vi "DAQmx 9411 6ch Digital Input (SubVI).vi"(0 "9411 Name":tag="9411", 11 "Error Input":errorcluster) -> (4 "Digital Inputs":bool[](array[boolean]), 15 "9411 Error":errorcluster)   [LabVIEW 2012]
uses:
  <vilib>/DAQmx/read.llb/DAQmx Read (Digital 1D Bool NChan 1Samp 1Line).vi
  <vilib>/DAQmx/miscellaneous.llb/DAQmx Fill In Error Info.vi
  <vilib>/DAQmx/create/channels.llb/DAQmx Create Channel (DI-Digital Input).vi
panel:
  # "DAQmx - 9411\n6ch Digital Input\nCreated by Blake Otting 2011\nUpdated 2-19-2013"
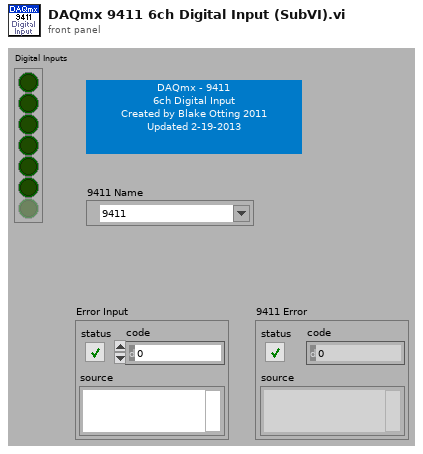
[diagram p1: front panel]
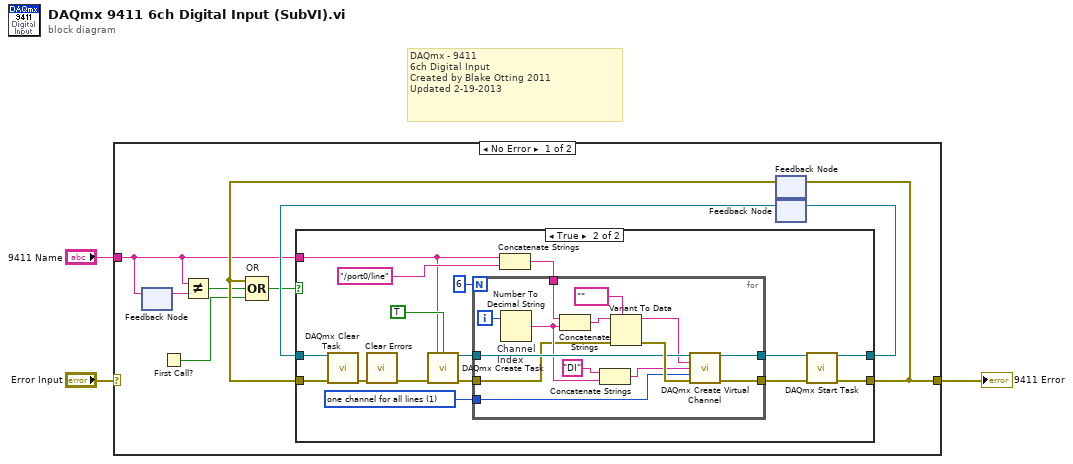
[diagram p0: block diagram]
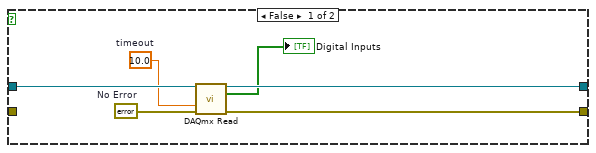
[diagram p2: hidden frame]
diagram:
  # "DAQmx - 9411\n6ch Digital Input\nCreated by Blake Otting 2011\nUpdated 2-19-2013"
  n1 = case shown="No Error" "Error Input" {
    selector: "Error Input" -> [_ w49]
    tunnel: "9411 Name" -> [w8 _]
    tunnel: [w4 w49] -> w2
    frame No Error {
      n2 = feedback #1() -> (w9:tag)  [unwired: 1 in]
      n3 = feedback-in #1(w8) -> ()
      n4 = First Call?() -> (First Call?: T/F=w6:bool)
      n5 = Not Equal?(x=w8, y=w9) -> (x != y?=w7:bool)
      n6 = feedback #2() -> (w10:errorcluster)  [unwired: 1 in]
      n7 = Compound Arithmetic op=OR "OR"(w10, w7, w6) -> (w5:bool)
      n8 = feedback #3() -> (w11:refnum<k21>)  [unwired: 1 in]
      n9 = case shown="True" w5 {
        tunnel: [w17 w30] -> w12
        tunnel: [w16 w29] -> w4
        tunnel: w10 -> [_ w33]
        tunnel: w11 -> [w18 w32]
        tunnel: w8 -> [_ w22]
        frame False {
          w13 = errorcluster {"status"=FALSE, "code"=0, "source"=""}  # No Error
          w15 = 10.0  # timeout
          n10 = call-poly <vilib>:"DAQmx Read.vi"("task/channels in"=w18, "timeout"=w15, "error in"=w13) -> ("task out"=w17:refnum<k21>, "data"=→"Digital Inputs":bool[], "error out"=w16:errorcluster)  [unwired: 10 in]
        }
        frame True {
          w24 = 1 items=["one channel for each line", "one channel for all lines"] ("line grouping")
          n11 = call <vilib>:"DAQmx Clear Task.vi"("task in"=w32, "error in"=w33) -> ("error out"=w20:errorcluster)  [unwired: 13 in]
          n12 = call <vilib>:"Clear Errors.vi"("error in (no error)"=w20) -> ("error out"=w21:errorcluster)  [unwired: 6 in]
          n13 = call <vilib>:"DAQmx Create Task.vi"("new task name"=w22, "auto cleanup"=TRUE, "error in"=w21) -> ("task out"=w27:refnum<k21>, "error out"=w25:errorcluster)  [unwired: 11 in]
          n14 = Concatenate Strings(w22, "/port0/line" ("physical channel")) -> (w26:string)
          n15 = for {
            N: 6 -> [_]
            tunnel: w26 -> [w47]
            tunnel: [w42] -> w23
            tunnel: w27 -> [w44]
            tunnel: [w43] -> w19
            tunnel: w25 -> [w36]
            tunnel: w24 -> [w35]
            i -> [w48]
            n16 = Number To Decimal String "Channel\nIndex"(number=w48) -> (decimal integer string=w39:string)  [unwired: 1 in]
            n17 = Concatenate Strings(w47, w39) -> (w45:string)
            n18 = Concatenate Strings("DI", w39) -> (w37:string)
            n19 = Variant To Data(error in=w36, type=tag "", Variant=w45) -> (data=w40:tag, error out=w46:errorcluster)
            n20 = call-poly <vilib>:"DAQmx Create Virtual Channel.vi"("task in"=w44, "lines"=w40, "name to assign"=w37, "line grouping"=w35, "error in"=w46) -> ("task out"=w43:refnum<k21>, "error out"=w42:errorcluster)  [unwired: 9 in]
          }
          n21 = call <vilib>:"DAQmx Start Task.vi"("task/channels in"=w19, "error in"=w23) -> ("task out"=w30:refnum<k21>, "error out"=w29:errorcluster)  [unwired: 12 in]
        }
      }
      n22 = feedback-in #2(w4) -> ()
      n23 = feedback-in #3(w12) -> ()
    }
    frame Error {
    }
  }
  "9411 Error" <- w2
